vi "Close_RESTful_connection.vi"(8 "error in (no error)":errorcluster, 11 "REST Client in":refnum<class "REST Client.lvclass">) -> (0 "error out":errorcluster)   [LabVIEW 2024]
uses:
  <vilib>/addons/_JKI.lib/REST Client/classes/REST Client/REST Client.lvclass
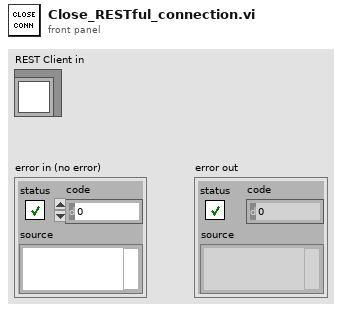
[diagram p1: front panel]
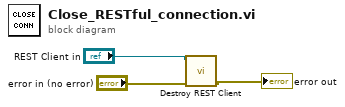
[diagram p0: block diagram]
diagram:
  n1 = call-dynamic "Destroy REST Client.vi"("error in (no error)"="error in (no error)", "REST Client in"="REST Client in") -> ("error out"=→"error out":errorcluster)  [unwired: 9 in]
